vi "Initialize Hardware.vi"(8 "error in (no error)":errorcluster, 9 "Connection Ref":variant, 10 "DAQ Type":enum16{"Hardware", "Simulation"}(ring), 11 "ARS-0220 in":refnum<class "ARS-0220.lvclass">) -> (0 "error out":errorcluster, 3 "ARS-0220 out":refnum<class "ARS-0220.lvclass">)   [LabVIEW 2021, in "Environment Chamber.lvlib" / "ARS-0220.lvclass"]
uses:
  ARS-0220.lvclass
  ARS-0220.lvclass/ARS-0220.ctl
  Support Libraries/Climatic Chamber/Climatic Chamber.lvlib
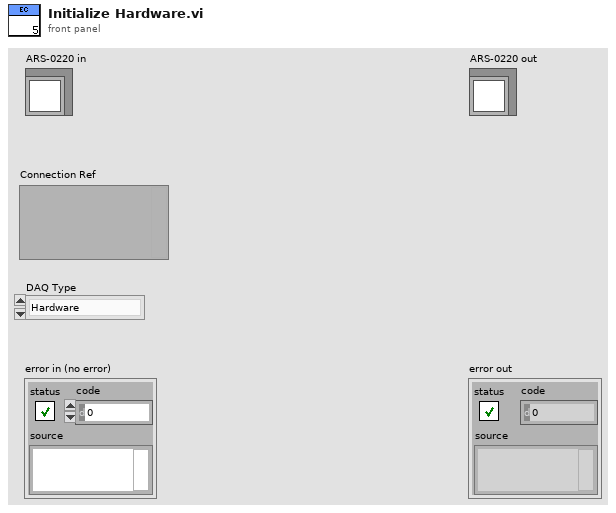
[diagram p1: front panel]
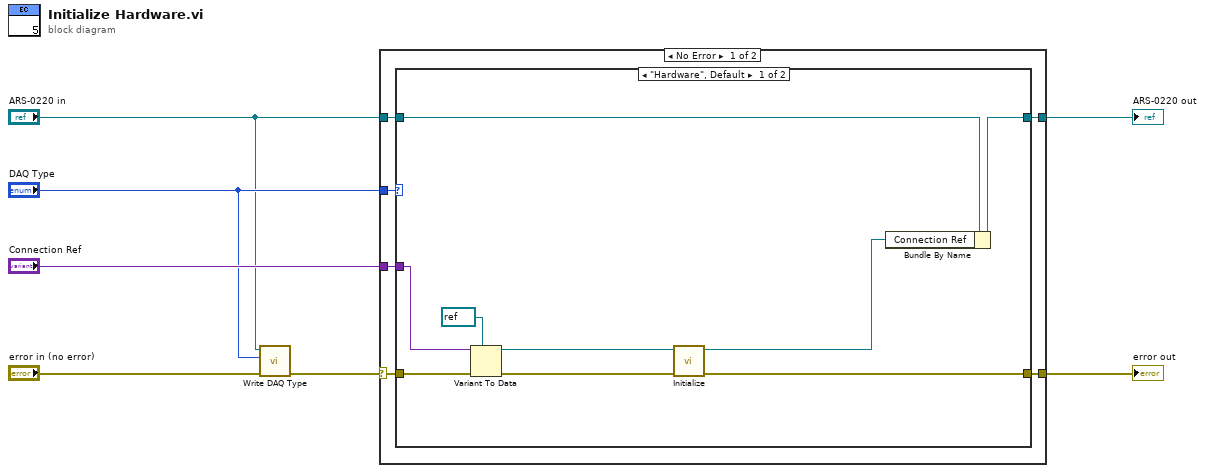
[diagram p0: block diagram]
diagram:
  n1 = call "Write DAQ Type.vi"("error in (no error)"="error in (no error)", "DAQ Type"="DAQ Type", "ARS-0220 in"="ARS-0220 in") -> ("error out"=w6:errorcluster)  [unwired: 7 in, 1 out]
  n2 = case shown="No Error" w6 {
    selector: w6 -> [w10 w25]
    tunnel: "DAQ Type" -> [w12 _]
    tunnel: "ARS-0220 in" -> [w13 w26]
    tunnel: "Connection Ref" -> [w11 _]
    tunnel: [w9 w25] -> w2
    tunnel: [w8 w26] -> w1
    frame No Error {
      n3 = case shown="\"Hardware\", Default" w12 {
        tunnel: w13 -> [w16 w24]
        tunnel: w11 -> [w20 _]
        tunnel: w10 -> [w22 w23]
        tunnel: [w17 w23] -> w9
        tunnel: [w15 w24] -> w8
        frame "Hardware", Default {
          n4 = Variant To Data(error in=w22, type=refnum<visa-resource-name> refnum ("VISA resource name"), Variant=w20) -> (data=w18:refnum<visa-resource-name>, error out=w21:errorcluster)
          n5 = call "Initialize.vi"("error in (no error)"=w21, "VISA resource name"=w18) -> ("error out"=w17:errorcluster, "VISA resource name out"=w14:refnum<visa-resource-name>)  [unwired: 8 in]
          n6 = Bundle By Name(cluster=w16, "Connection Ref"=w14) -> (w15:refnum<class "ARS-0220.lvclass">)
        }
        frame "Simulation" {
        }
      }
    }
    frame Error {
    }
  }
  "error out" <- w2
  "ARS-0220 out" <- w1
